vi "LWXPS_PositionerCorrectorNotchFiltersSet.vi"(0 "Notch Frequency 1":dbl, 1 "Positioner Name":string, 2 "XPS Reference IN":refnum<k24>, 5 "Notch Bandwidth 1":dbl, 7 "Notch Gain 1":dbl, 9 "Notch Frequency 2":dbl, 11 "Notch Bandwidth 2":dbl, 12 "Notch Gain 2":dbl, 13 "LabVIEW error IN":errorcluster) -> (4 "XPS Reference OUT":refnum<k24>, 6 "Returned error code":i32, 10 "XPS Error String":string, 15 "LabVIEW error OUT":errorcluster)   [LabVIEW 2014]
uses:
  D:/XPSQ8_LabView_Library/Development/Source/Dll/Newport.XPS.CommandInterface.dll
  Dll/Newport.XPS.CommandInterface.dll
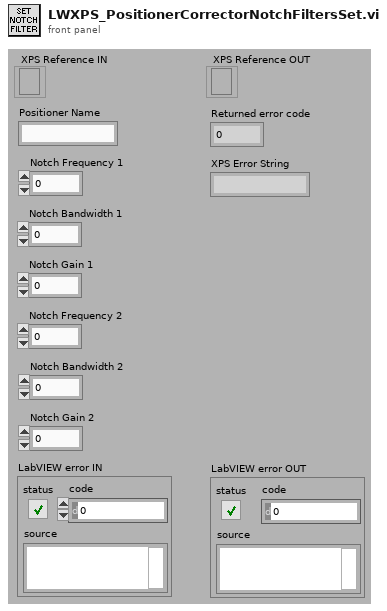
[diagram p1: front panel]
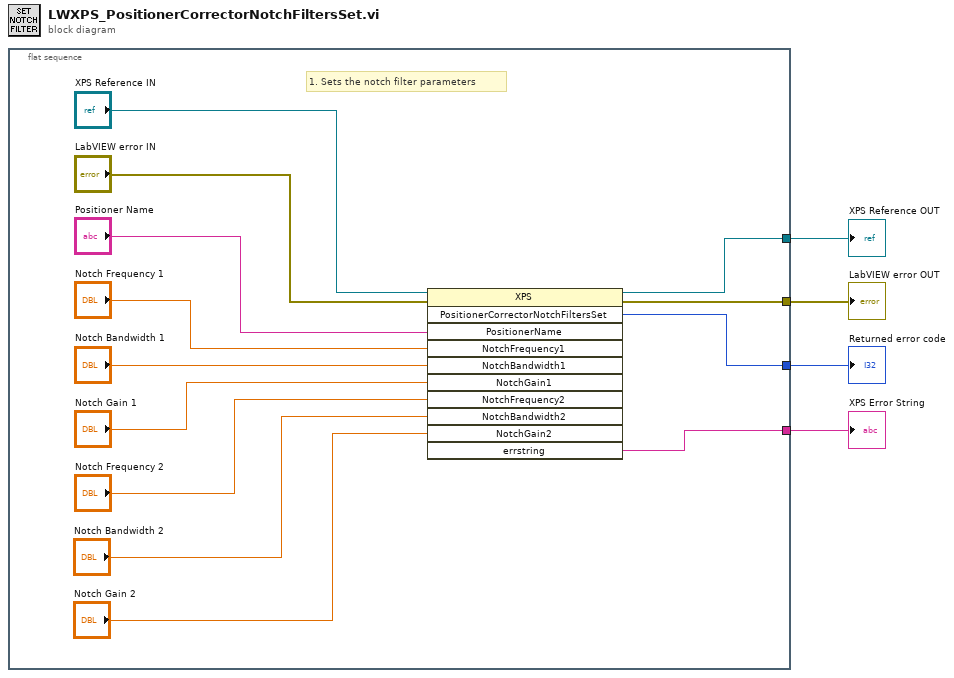
[diagram p0: block diagram]
diagram:
  n1 = flat-sequence {
    tunnel: [w15] -> w4
    tunnel: [w14] -> w3
    tunnel: [w16] -> w2
    tunnel: [w5] -> w1
    frame #0 {
      # "1. Sets the notch filter parameters"
      n2 = invoke class="XPS" method="PositionerCorrectorNotchFiltersSet"(reference="XPS Reference IN", error in="LabVIEW error IN", "PositionerName"="Positioner Name", "NotchFrequency1"="Notch Frequency 1", "NotchBandwidth1"="Notch Bandwidth 1", "NotchGain1"="Notch Gain 1", "NotchFrequency2"="Notch Frequency 2", "NotchBandwidth2"="Notch Bandwidth 2", "NotchGain2"="Notch Gain 2") -> (reference out=w15:refnum<k24>, error out=w14:errorcluster, "PositionerCorrectorNotchFiltersSet"=w16:i32, "errstring"=w5:string)  [unwired: 2 in, 7 out]
    }
  }
  "XPS Error String" <- w1
  "XPS Reference OUT" <- w4
  "LabVIEW error OUT" <- w3
  "Returned error code" <- w2
